vi "LR-Extinction-time.vi"(5 "Test characteristics":T2, 7 "Extinction time settings":T4={"Treshold [%]"=80}, 8 "error in (no error)":errorcluster, 9 "Power in":dbl[](array[numeric]), 11 "Results in":T1) -> (0 "error out":errorcluster, 1 "Power":dbl[](array[numeric]), 3 "Results":T1, 4 "Valid?":bool)   [LabVIEW 2013, in "HardwareCharacterization.lvlib" / "HC-LaserResponse.lvclass"]
doc: "Use this template to build a VI to use as a subVI."
uses:
  HC-LaserResponse.lvclass
  Settings-extinction.ctl
  Test-characteristics.ctl
  Detectors.ctl
  Test-results.ctl
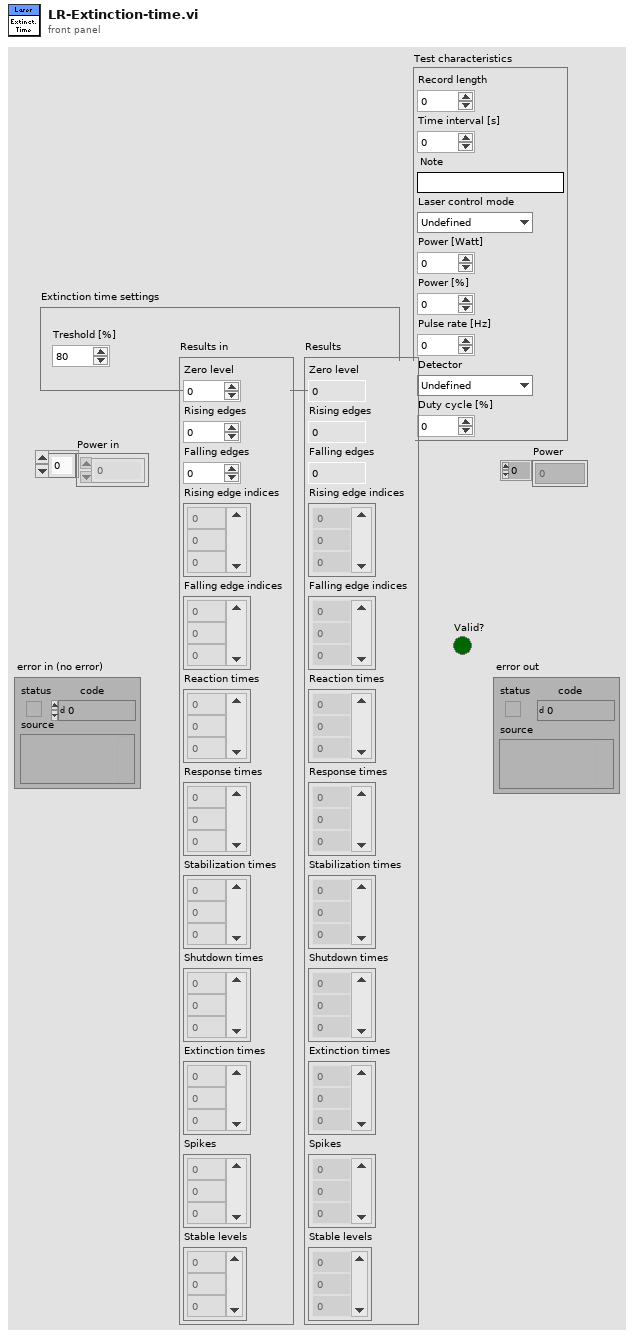
[diagram p1: front panel]
types:
  T1 = typedef "HardwareCharacterization.lvlib/HC-LaserResponse.lvclass/Test-results.ctl" = cluster{"Zero level":dbl, "Rising edges":i32, "Falling edges":i32, "Rising edge indices":dbl[], "Falling edge indices":dbl[], "Reaction times":dbl[], "Response times":dbl[], "Stabilization times":dbl[], "Shutdown times":dbl[], "Extinction times":dbl[], "Spikes":i32[], "Stable levels":dbl[]}
  T2 = typedef "HardwareCharacterization.lvlib/HC-LaserResponse.lvclass/Test-characteristics.ctl" = cluster{"Record length":i32, "Time interval [s]":dbl, "Note":string, "Laser control mode":enum16{"Undefined", "Modulation (digital)", "Power variation (analog)"}, "Power [Watt]":dbl, "Power [%]":dbl, "Pulse rate [Hz]":dbl, "Detector":T3, "Duty cycle [%]":dbl}
  T3 = typedef "HardwareCharacterization.lvlib/HC-LaserResponse.lvclass/Detectors.ctl" = enum16{"Undefined", "DET10A", "DET10A - 2kOhm ", "PDA36A - 0dB"}
  T4 = typedef "HardwareCharacterization.lvlib/HC-LaserResponse.lvclass/Settings-extinction.ctl" = cluster{"Treshold [%]":i32}
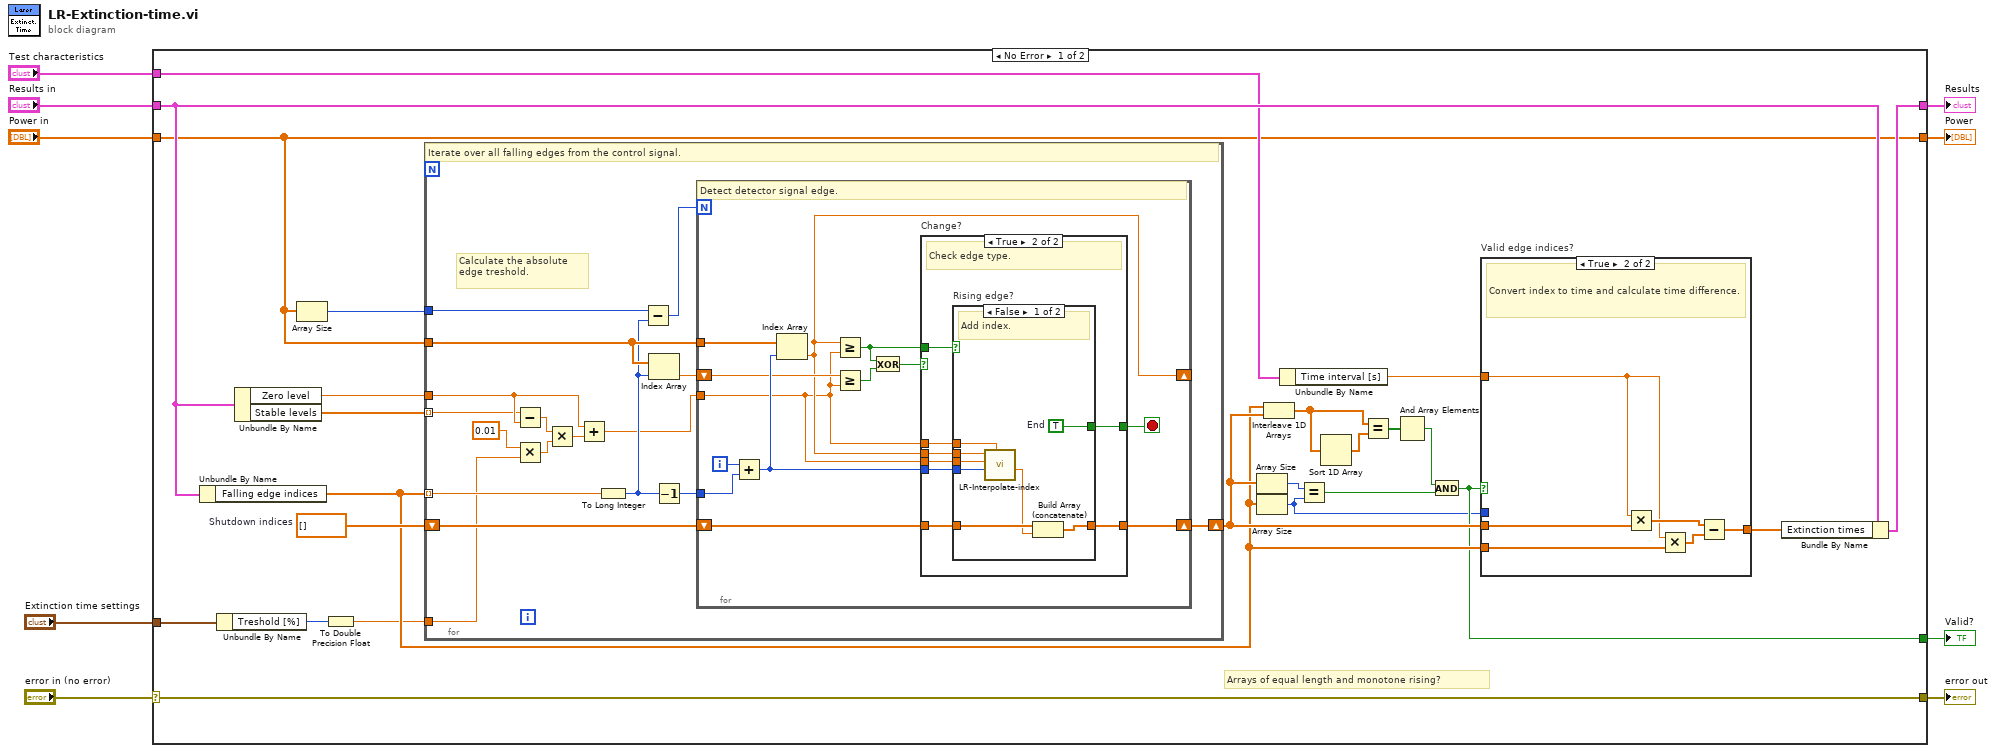
[diagram p0: block diagram]
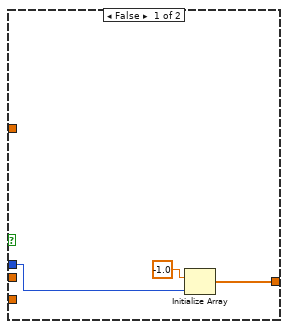
[diagram p2: hidden frame]
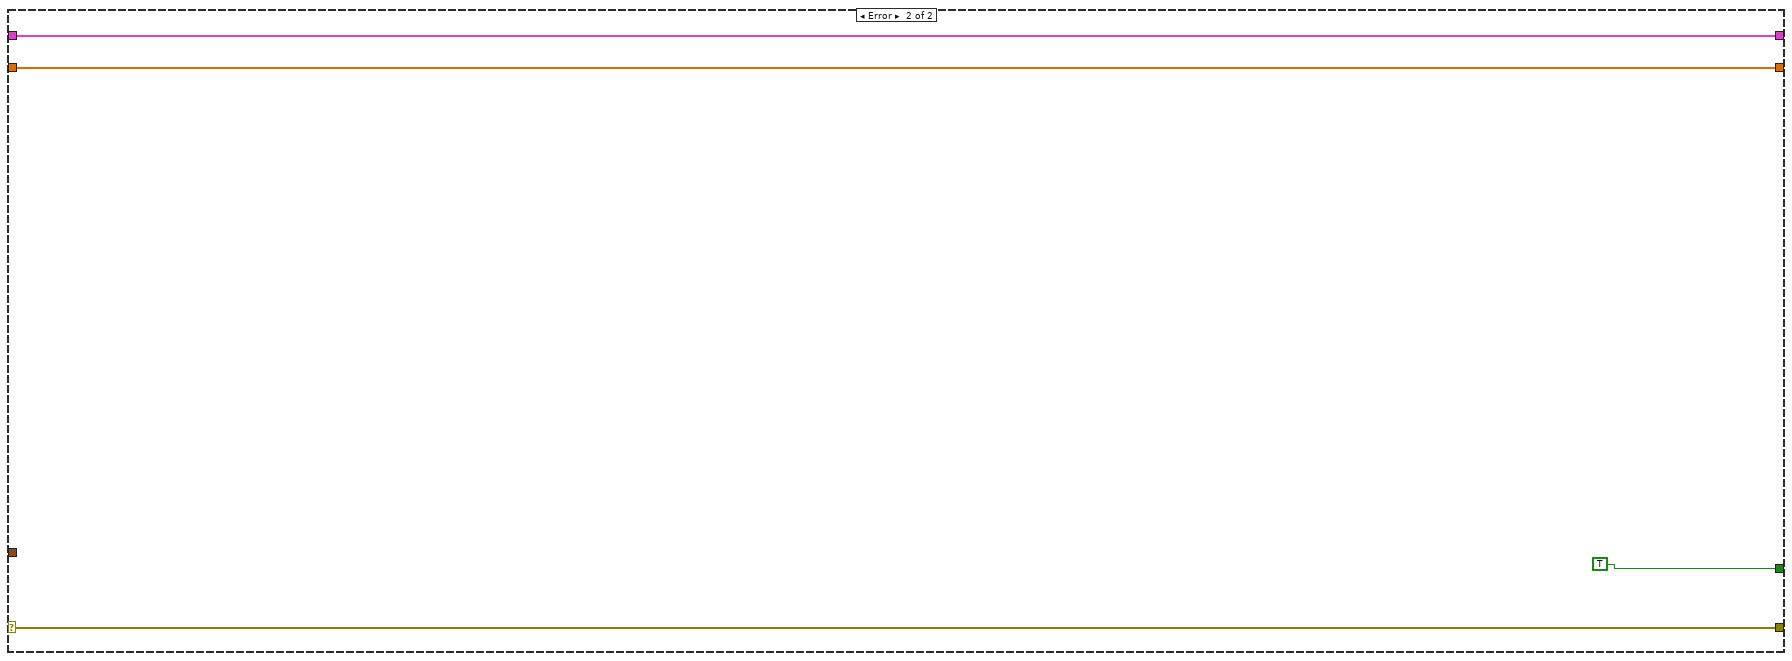
[diagram p5: hidden frame]
diagram:
  n1 = case shown="No Error" "error in (no error)" {
    selector: "error in (no error)" -> [w31 w94]
    tunnel: [w31 w94] -> w9
    tunnel: "Results in" -> [w26 w93]
    tunnel: "Extinction time settings" -> [w33 _]
    tunnel: [w20 TRUE] -> w8
    tunnel: [w27 w93] -> w2
    tunnel: "Power in" -> [w14 w91]
    tunnel: "Test characteristics" -> [w16 _]
    tunnel: [w14 w91] -> w1
    frame No Error {
      w32 = dbl[] []  # Shutdown indices
      # "Arrays of equal length and monotone rising?"
      n2 = Unbundle By Name(w26) -> ("Falling edge indices"=w21:dbl[])
      n3 = Unbundle By Name(w33) -> ("Treshold [%]"=w13:i32)
      n4 = Unbundle By Name(w26) -> ("Zero level"=w11:dbl, "Stable levels"=w10:dbl[])
      n5 = Array Size(array=w14) -> (size(s)=w18:i32)
      n6 = To Double Precision Float(number=w13) -> (double precision float=w12:dbl)
      n7 = for {
        tunnel: w14 -> [w54]
        tunnel: w21 -> [w53] mode=indexing
        shift-right: [w58] -> w22
        shift-left: w32 -> [w59]
        tunnel: w18 -> [w56]
        tunnel: w12 -> [w46]
        tunnel: w11 -> [w44]
        tunnel: w10 -> [w43] mode=indexing
        # "Calculate the absolute\nedge treshold."
        # "Iterate over all falling edges from the control signal."
        n8 = Subtract(x=w43, y=w44) -> (x-y=w48:dbl)
        n9 = Multiply(x=0.01, y=w46) -> (x*y=w49:dbl)
        n10 = Multiply(x=w48, y=w49) -> (x*y=w47:dbl)
        n11 = Add(x=w44, y=w47) -> (x+y=w45:dbl)
        n12 = To Long Integer(number=w53) -> (32bit integer=w51:i32)
        n13 = Subtract(x=w56, y=w51) -> (x-y=w55:i32)
        n14 = Index Array(array=w54, index=w51) -> (element=w52:dbl)
        n15 = Decrement(x=w51) -> (x-1=w57:i32)
        n16 = for {
          N: w55 -> [_]
          tunnel: w54 -> [w66]
          tunnel: w45 -> [w60]
          shift-right: [w68] -> w58
          shift-left: w59 -> [w69]
          shift-right: [w61] -> _
          shift-left: w52 -> [w62]
          tunnel: w57 -> [w65]
          i -> [w67]
          stop <- w63 stop-if-true
          # "Detect detector signal edge."
          n17 = Add(x=w67, y=w65) -> (x+y=w64:i32)
          n18 = Index Array(array=w66, index=w64) -> (element=w61:dbl)
          n19 = Greater Or Equal?(x=w61, y=w60) -> (x >= y?=w70:bool)
          n20 = Greater Or Equal?(x=w62, y=w60) -> (x >= y?=w71:bool)
          n21 = Exclusive Or(1:w71, 2:w70) -> (0:w72:bool)
          n22 = case "Change?" shown="True" w72 {
            tunnel: w70 -> [_ w81]
            tunnel: w69 -> [w73 w80]
            tunnel: w64 -> [_ w79]
            tunnel: [w73 w78] -> w68
            tunnel: [_ w77] -> w63
            tunnel: w61 -> [_ w76]
            tunnel: w60 -> [_ w75]
            tunnel: w60 -> [_ w74]
            frame False {
              # "Do nothing."
            }
            frame True {
              # "Check edge type."
              n23 = case "Rising edge?" shown="False" w81 {
                tunnel: w80 -> [w89 w90]
                tunnel: w79 -> [w85 _]
                tunnel: [w88 w90] -> w78
                tunnel: [w87 _] -> w77
                tunnel: w76 -> [w84 _]
                tunnel: w75 -> [w83 _]
                tunnel: w74 -> [w82 _]
                frame False {
                  w87 = TRUE  # End
                  # "Add index."
                  n24 = call "LR-Interpolate-index.vi"("Value"=w82, "Lower index"=w85, "Previous"=w83, "Current"=w84) -> ("Fractional index"=w86:dbl)  [unwired: 6 in, 1 out]
                  n25 = Build Array (concatenate)(w89, w86) -> (w88:dbl[])
                }
                frame True {
                  # "Do nothing."
                }
              }
            }
          }
        }
      }
      n26 = Array Size(array=w22) -> (size(s)=w25:i32)
      n27 = Array Size(array=w21) -> (size(s)=w17:i32)
      n28 = Interleave 1D Arrays(w21, w22) -> (w30:dbl[])
      n29 = Unbundle By Name(w16) -> ("Time interval [s]"=w15:dbl)
      n30 = Equal?(x=w25, y=w17) -> (x = y?=w23:bool)
      n31 = Sort 1D Array(array=w30) -> (sorted array=w29:dbl[])
      n32 = Equal?(x=w30, y=w29) -> (x = y?=w28:bool[])
      n33 = And Array Elements(Boolean array=w28) -> (logical AND=w24:bool)
      n34 = And(x=w24, y=w23) -> (x .and. y?=w20:bool)
      n35 = case "Valid edge indices?" shown="True" w20 {
        tunnel: w22 -> [_ w39]
        tunnel: w21 -> [_ w38]
        tunnel: [w34 w40] -> w19
        tunnel: w17 -> [w35 _]
        tunnel: w15 -> [_ w37]
        frame False {
          n36 = Initialize Array(-1.0, w35) -> (w34:dbl[])
        }
        frame True {
          # "Convert index to time and calculate time difference."
          n37 = Multiply(x=w37, y=w39) -> (x*y=w41:dbl[])
          n38 = Multiply(x=w37, y=w38) -> (x*y=w42:dbl[])
          n39 = Subtract(x=w41, y=w42) -> (x-y=w40:dbl[])
        }
      }
      n40 = Bundle By Name(cluster=w26, "Extinction times"=w19) -> (w27:T1)
    }
    frame Error {
    }
  }
  "Results" <- w2
  "error out" <- w9
  "Valid?" <- w8
  "Power" <- w1
